vi "ProblemasMonitoreo.vi"() -> ()   [LabVIEW 2020]
uses:
  <vilib>/Instr/_visa.llb/VISA Configure Serial Port (Instr).vi
panel:
  in  "Escribir datos":bool
  in  "stop":bool
  out "Datos enviados":string
  in  "Datos a enviar":string
  out "Serial Monitor":string
  in  "Leer datos":bool
  in  "COM Entrada":refnum<visa-resource-name>
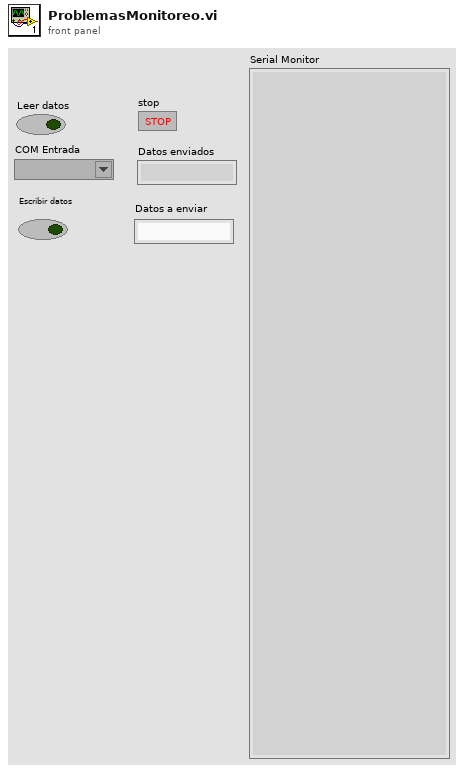
[diagram p1: front panel]
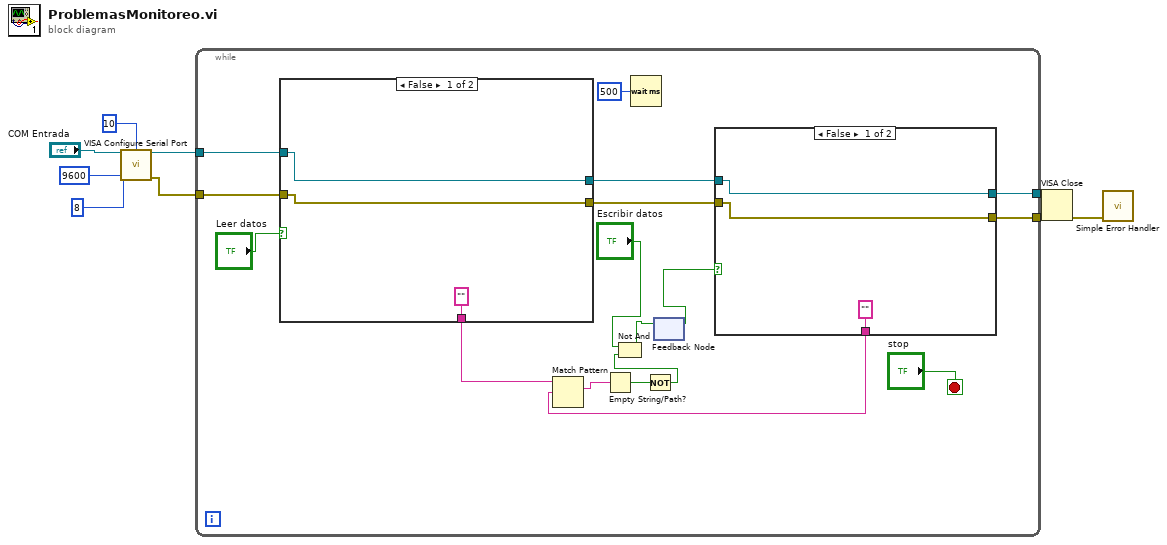
[diagram p0: block diagram]
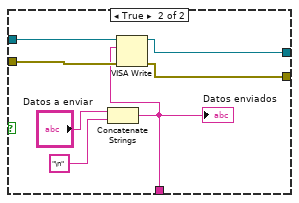
[diagram p2: hidden frame]
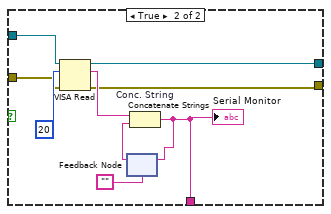
[diagram p3: hidden frame]
diagram:
  n1 = call-poly "VISA Configure Serial Port"("VISA resource name"="COM Entrada", "termination char\n(0xA = '\\n' = LF)"=u8 10 ("termination char\n(0xA = '\\n' = LF)"), "baud rate (9600)"=u32 9600, "data bits (8)"=u16 8) -> ("VISA resource name out"=w9:refnum<visa-resource-name>, "error out"=w5:errorcluster)  [unwired: 10 in]
  n2 = while {
    tunnel: w9 -> [w25]
    tunnel: w5 -> [w24]
    tunnel: [w20] -> w4
    tunnel: [w19] -> w3
    stop <- "stop" stop-if-true
    n3 = case shown="False" "Leer datos" {
      tunnel: w25 -> [w39 w47]
      tunnel: w24 -> [w38 w46]
      tunnel: [w39 w42] -> w22
      tunnel: [w38 w41] -> w21
      tunnel: ["" w40] -> w17
      frame False {
      }
      frame True {
        n4 = VISA Read(VISA resource name=w47, byte count=u32 20, error in (no error)=w46) -> (VISA resource name out=w42:refnum<visa-resource-name>, read buffer=w45:string, error out=w41:errorcluster)  [unwired: 1 out]
        n5 = feedback #1("") -> (w44:string)
        n6 = Concatenate Strings "Conc. String"(w45, w44) -> (w40:string)
        "Serial Monitor" <- w40
        n7 = feedback-in #1(w40) -> ()
      }
    }
    n8 = Wait (ms)(milliseconds to wait=u32 500) -> ()  [unwired: 1 out]
    n9 = feedback #2() -> (w10:bool)  [unwired: 1 in]
    n10 = case shown="False" w10 {
      tunnel: w22 -> [w29 w36]
      tunnel: w21 -> [w28 w35]
      tunnel: [w29 w32] -> w20
      tunnel: [w28 w31] -> w19
      tunnel: ["" w30] -> w16
      frame False {
      }
      frame True {
        n11 = Concatenate Strings("Datos a enviar", "\n" ("string")) -> (w30:string)
        "Datos enviados" <- w30
        n12 = VISA Write(VISA resource name=w36, write buffer=w30, error in (no error)=w35) -> (VISA resource name out=w32:refnum<visa-resource-name>, error out=w31:errorcluster)  [unwired: 1 out]
      }
    }
    n13 = Match Pattern(string=w17, regular expression=w16) -> (match substring=w15:string)  [unwired: 1 in, 3 out]
    n14 = Empty String/Path?(string/path=w15) -> (empty?=w14:bool)
    n15 = Not(x=w14) -> (.not. x?=w12:bool)
    n16 = Not And(1:w12, 2:"Escribir datos") -> (0:w11:bool)
    n17 = feedback-in #2(w11) -> ()
  }
  n18 = VISA Close(VISA resource name=w4, error in (no error)=w3) -> (error out=w2:errorcluster)
  n19 = call <vilib>:"Simple Error Handler.vi"("error in (no error)"=w2) -> ()  [unwired: 4 in, 5 out]
